vi "Convert FPGA Refnum to Session.vi"(8 "error in (no error)":errorcluster, 11 "fpga refnum in":refnum<k20>) -> (0 "error out":errorcluster, 3 "session out":u64)   [LabVIEW 2020, in "FPGA Register IO.lvlib"]
uses:
  FPGA Register IO.lvlib
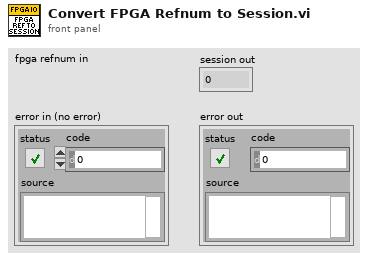
[diagram p1: front panel]
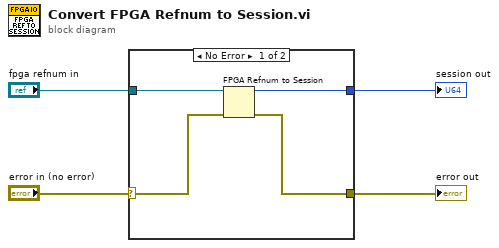
[diagram p0: block diagram]
diagram:
  n1 = case shown="No Error" "error in (no error)" {
    selector: "error in (no error)" -> [w5 w9]
    tunnel: [w8 _] -> w4
    tunnel: [w7 w9] -> w3
    tunnel: "fpga refnum in" -> [w6 _]
    frame No Error {
      n2 = FPGA Refnum to Session(4:w5, 7:w6) -> (0:w7:errorcluster, 3:w8:u64)
    }
    frame Error {
    }
  }
  "session out" <- w4
  "error out" <- w3
